vi "Search for oldest time to keep DBL.vi"(9 "oldest time to keep":dbl, 11 "timestamps (incrementing)":dbl[](array[numeric])) -> (1 "split index":i32, 3 "timestamps (dup)":dbl[](array[numeric]))   [LabVIEW 2021, in "RocketPlot.lvlib"]
uses:
  RocketPlot.lvlib
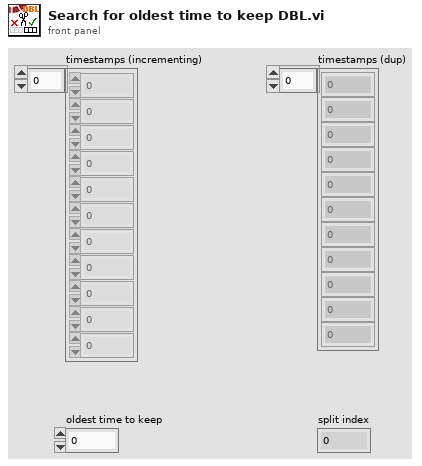
[diagram p1: front panel]
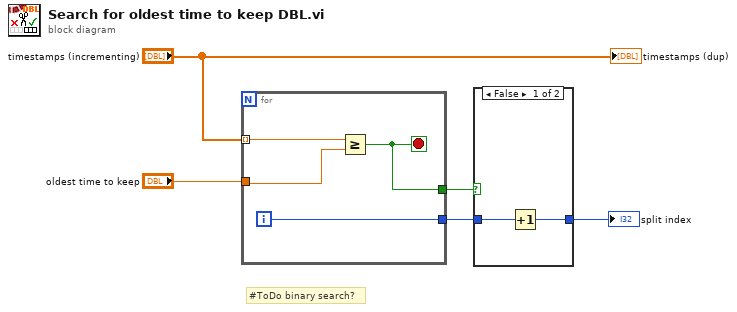
[diagram p0: block diagram]
diagram:
  # "#ToDo binary search?"
  n1 = for {
    tunnel: "timestamps (incrementing)" -> [w9] mode=indexing
    tunnel: "oldest time to keep" -> [w8]
    tunnel: [w7] -> w4
    tunnel: [w6] -> w5
    i -> [w7]
    stop <- w6 stop-if-true
    n2 = Greater Or Equal?(x=w9, y=w8) -> (x >= y?=w6:bool)
  }
  n3 = case shown="False" w5 {
    tunnel: w4 -> [w11 w12]
    tunnel: [w10 w12] -> w3
    frame False {
      n4 = Increment(x=w11) -> (x+1=w10:i32)
    }
    frame True {
    }
  }
  "split index" <- w3
  "timestamps (dup)" <- "timestamps (incrementing)"
